vi "Motion Profile Run.vi"(6 "Synchronication":enum16{"Start", "Wait"}(ring)=enum."Wait", 7 "Description":string, 8 "Command Info In":T1, 11 "Duration":dbl) -> (0 "Command Info Out":T1)   [LabVIEW 2017]
doc: "This VI notifies the subsystem to perform this command for the given duration, then go back to the default state. Synchronization determines whether this VI Starts the operation and returns immediately, or waits for the operation to complete. The first option is commonly used for TeleOp, and the second for Autonomous sequencing."
uses:
  <vilib>/Rock Robotics/WPI/Framework/Command Status Info.ctl
  <vilib>/Rock Robotics/WPI/Framework/Completion Status.ctl
  <vilib>/Rock Robotics/WPI/Framework/Completion Notifier.ctl
  Implementation/Drive Setpoints.ctl
  Implementation/Drive Operations.ctl
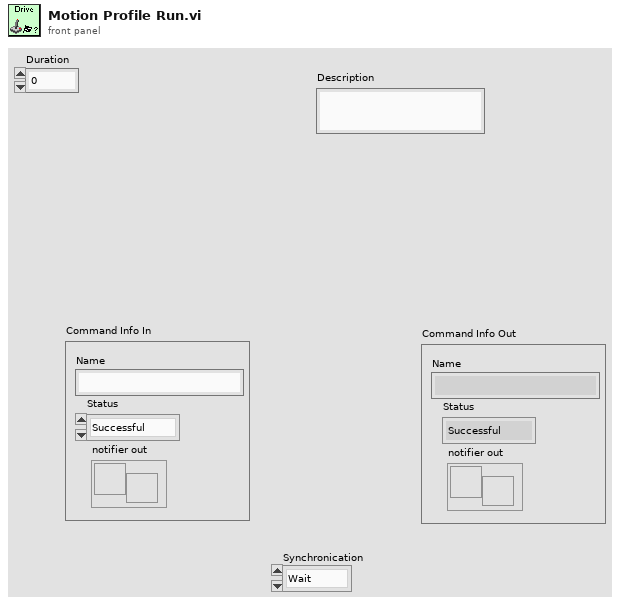
[diagram p1: front panel]
types:
  T1 = typedef "Command Status Info.ctl" = cluster{"Name":string, "Status":T2, "notifier out":T3}
  T2 = typedef "Completion Status.ctl" = enum16{"Successful", "Aborted", "Incomplete"}
  T3 = typedef "Completion Notifier.ctl" = refnum<notifier>
  T4 = typedef "Drive Setpoints.ctl" = cluster{"Operation":T5, "X Setpoint":dbl, "Y Setpoint":dbl, "Duration":dbl, "Z Setpoint":dbl, "Tracks":bool, "Gyro":dbl, "POV":i16, "Distance(feet)":dbl, "AutoTrack Toggle":bool, "Collsision Detection":bool, "Reset Encoder":bool, "MP File Name":string}
  T5 = typedef "Drive Operations.ctl" = enum16{"Reserve", "Read Current", "Reset Motors VBus", "Motion Profile run", "Immediate Robot Centric", "Drive for Time Robot Centric", "Immediate Field Centric", "Drive For Time Field Centric", "Button Adjust", "Set Motors Motion Profile", "Reset Encoders", "Drive for Distance"}
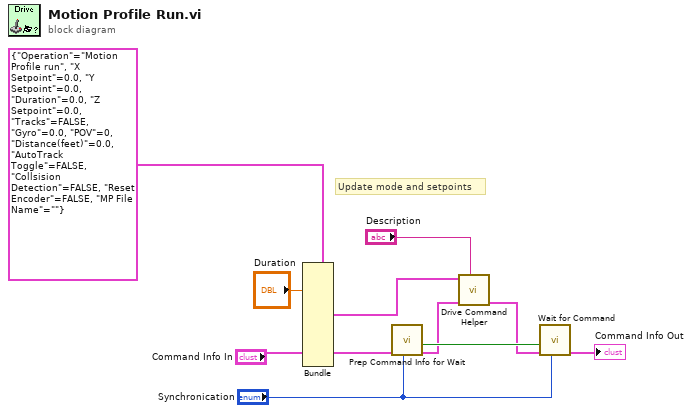
[diagram p0: block diagram]
diagram:
  # "Update mode and setpoints"
  n1 = Bundle(cluster=T4 {"Operation"=enum."Motion Profile run", "X Setpoint"=0.0, "Y Setpoint"=0.0, "Duration"=0.0, "Z Setpoint"=0.0, "Tracks"=FALSE, "Gyro"=0.0, "POV"=0, "Distance(feet)"=0.0, "AutoTrack Toggle"=FALSE, "Collsision Detection"=FALSE, "Reset Encoder"=FALSE, "MP File Name"=""} ("SubSystem Data"), "Duration"="Duration") -> (w3:T4)  [unwired: 12 in]
  n2 = call <vilib>:"Prep Command Info for Wait.vi"("Synchronication"="Synchronication", "Command Info"="Command Info In") -> ("Command Info"=w7:T1, "Allocated"=w8:bool)  [unwired: 8 in]
  n3 = call "Drive Command Helper.vi"("Description"="Description", "Command Info In"=w7, "SubSystem Data"=w3) -> ("Command Info Out"=w4:T1)  [unwired: 7 in, 1 out]
  n4 = call <vilib>:"Wait for Command.vi"("Synchronication"="Synchronication", "Command Info in"=w4, "Allocated"=w8) -> ("Command Info out"=→"Command Info Out":T1)  [unwired: 8 in]
